vi "Robot Main.vi"() -> ()   [LabVIEW 2019]
doc: "This VI implements the framework and scheduler for your robotics program. It should not be necessary to modify the framework. You are expected to add your code to the VIs called from Robot Main - the ones located in the Team Code folder within the project."
uses:
  <vilib>/Rock Robotics/SystemInterfaces/i2clib/i2c_bus.ctl
panel:
  out "Normalized \nMeasured\nColor":cluster{"R":dbl, "G":dbl, "B":dbl}
  in  "UpdateColors":bool
  in  "Update Blue \nCalibration":cluster{"R":dbl, "G":dbl, "B":dbl}={"R"=0.143, "G"=0.427, "B"=0.429}
  in  "Update Green \nCalibration":cluster{"R":dbl, "G":dbl, "B":dbl}={"R"=0.197, "G"=0.561, "B"=0.24}
  in  "Update Red \nCalibration":cluster{"R":dbl, "G":dbl, "B":dbl}={"R"=0.561, "G"=0.323, "B"=0.114}
  in  "Update Yellow \nCalibration":cluster{"R":dbl, "G":dbl, "B":dbl}={"R"=0.361, "G"=0.524, "B"=0.113}
  out "Matched Color Name":string
  out "Match Confidence":dbl
  out "Measured Color":cluster{"R":dbl, "G":dbl, "B":dbl}
  in  "Init Blue \nCalibration":cluster{"R":dbl, "G":dbl, "B":dbl}={"R"=0.143, "G"=0.427, "B"=0.429}
  in  "Init Green \nCalibration":cluster{"R":dbl, "G":dbl, "B":dbl}={"R"=0.197, "G"=0.561, "B"=0.24}
  in  "Init Red \nCalibration":cluster{"R":dbl, "G":dbl, "B":dbl}={"R"=0.561, "G"=0.323, "B"=0.114}
  in  "Init Yellow \nCalibration":cluster{"R":dbl, "G":dbl, "B":dbl}={"R"=0.361, "G"=0.524, "B"=0.113}
  out "error out":errorcluster
  out "Proximity":u16(graph)
  out "Color":u32(colorbox)
  in  "I2C Bus":T1
  in  "Finish":bool
  # "Set These Items before running\nprogram"
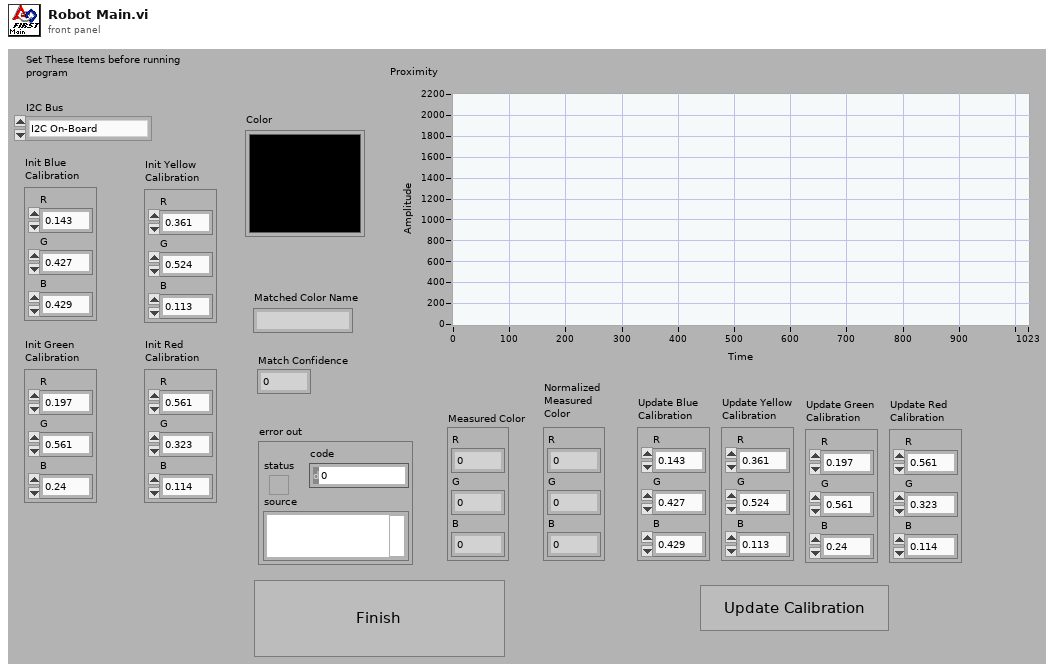
[diagram p1: front panel]
types:
  T1 = typedef "i2c_bus.ctl" = enum16{"I2C On-Board", "I2C MXP", "Invalid"}
  T2 = typedef "Color Sensor V3 DevRef.ctl" = cluster{"I2CDevRef":T3}
  T3 = typedef "WPI_I2CDevRef.ctl" = cluster{"DevStatus":errorcluster, "Device Address":u8, "Handle":i32, "I2C Bus":T1}
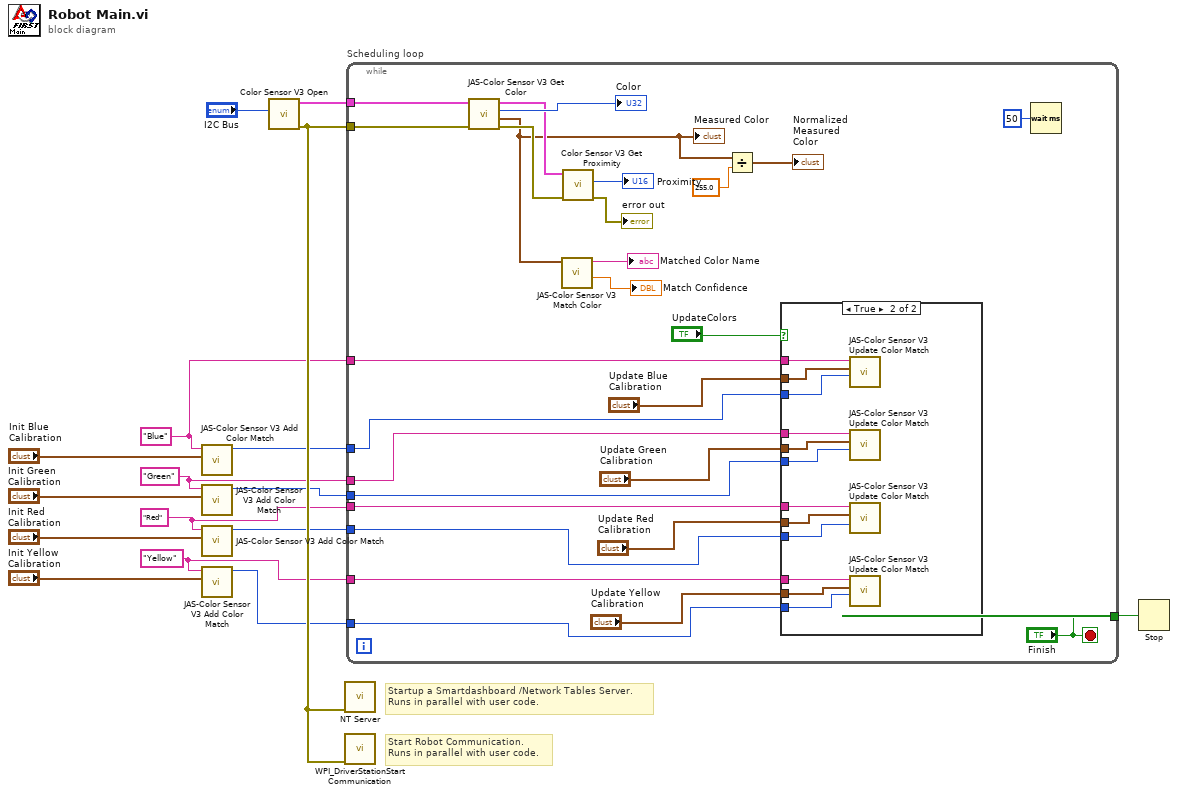
[diagram p0: block diagram]
diagram:
  w4 = "Yellow" ("Name")
  w5 = "Red" ("Name")
  w6 = "Green" ("Name")
  w7 = "Blue" ("Name")
  # "Startup a Smartdashboard /Network Tables Server.\nRuns in parallel with user code."
  # "Start Robot Communication.\nRuns in parallel with user code."
  n1 = call "JAS-Color Sensor V3 Add Color Match.vi"("Color"="Init Blue \nCalibration", "Name"=w7) -> ("ColorIndex"=w8:i32)  [unwired: 9 in]
  n2 = call "JAS-Color Sensor V3 Add Color Match.vi"("Color"="Init Green \nCalibration", "Name"=w6) -> ("ColorIndex"=w3:i32)  [unwired: 9 in]
  n3 = call "JAS-Color Sensor V3 Add Color Match.vi"("Color"="Init Red \nCalibration", "Name"=w5) -> ("ColorIndex"=w2:i32)  [unwired: 9 in]
  n4 = call "JAS-Color Sensor V3 Add Color Match.vi"("Color"="Init Yellow \nCalibration", "Name"=w4) -> ("ColorIndex"=w1:i32)  [unwired: 9 in]
  n5 = call <vilib>:"Color Sensor V3 Open.vi"("I2C Bus"="I2C Bus") -> ("error out"=w14:errorcluster, "ColorSensorDevRef"=w15:T2)  [unwired: 9 in]
  n6 = call <vilib>:"NT Server.vi"("error in (no error)"=w14) -> ()  [unwired: 11 in]
  n7 = call <vilib>:"WPI_DriverStationStart Communication.vi"("error in (no error)"=w14) -> ()  [unwired: 1 in, 10 out]
  n8 = while "Scheduling loop" {
    tunnel: w15 -> [w36]
    tunnel: w14 -> [w35]
    tunnel: ["Finish"] -> w13
    tunnel: w8 -> [w22]
    tunnel: w7 -> [w28]
    tunnel: w6 -> [w26]
    tunnel: w5 -> [w24]
    tunnel: w4 -> [w23]
    tunnel: w3 -> [w21]
    tunnel: w2 -> [w19]
    tunnel: w1 -> [w18]
    stop <- "Finish" stop-if-true
    n9 = call "JAS-Color Sensor V3 Get Color.vi"("error in (no error)"=w35, "ColorSensorDevRef"=w36) -> ("error out"=w41:errorcluster, "Normalized Color"=w32:cluster{"R":dbl, "G":dbl, "B":dbl}, "Color"=→"Color":u32, "ColorSensorDevRef out"=w40:T2)  [unwired: 6 in]
    "Measured Color" <- w32
    n10 = call "JAS-Color Sensor V3 Match Color.vi"("Measured Color"=w32) -> ("Confidence"=→"Match Confidence":dbl, "Matched Color Name"=→"Matched Color Name":string)  [unwired: 8 in, 1 out]
    n11 = call <vilib>:"Color Sensor V3 Get Proximity.vi"("error in (no error)"=w41, "ColorSensorDevRef"=w40) -> ("error out"=→"error out":errorcluster, "Proximity"=→"Proximity":u16)  [unwired: 7 in, 1 out]
    n12 = Divide(x=w32, y=255.0) -> (x/y=→"Normalized \nMeasured\nColor":cluster{"R":dbl, "G":dbl, "B":dbl})
    n13 = case shown="True" "UpdateColors" {
      tunnel: w28 -> [_ w55]
      tunnel: "Update Blue \nCalibration" -> [_ w54]
      tunnel: w26 -> [_ w53]
      tunnel: "Update Green \nCalibration" -> [_ w52]
      tunnel: w24 -> [_ w51]
      tunnel: w23 -> [_ w50]
      tunnel: w22 -> [_ w49]
      tunnel: w21 -> [_ w48]
      tunnel: "Update Red \nCalibration" -> [_ w47]
      tunnel: w19 -> [_ w46]
      tunnel: w18 -> [_ w44]
      tunnel: "Update Yellow \nCalibration" -> [_ w45]
      frame False {
      }
      frame True {
        n14 = call "JAS-Color Sensor V3 Update Color Match.vi"("ColorIndex"=w49, "Color"=w54, "Name"=w55) -> ()  [unwired: 9 in]
        n15 = call "JAS-Color Sensor V3 Update Color Match.vi"("ColorIndex"=w48, "Color"=w52, "Name"=w53) -> ()  [unwired: 9 in]
        n16 = call "JAS-Color Sensor V3 Update Color Match.vi"("ColorIndex"=w46, "Color"=w47, "Name"=w51) -> ()  [unwired: 9 in]
        n17 = call "JAS-Color Sensor V3 Update Color Match.vi"("ColorIndex"=w44, "Color"=w45, "Name"=w50) -> ()  [unwired: 9 in]
      }
    }
    n18 = Wait (ms)(milliseconds to wait=u32 50) -> ()  [unwired: 1 out]
  }
  n19 = Stop(stop? (T)=w13) -> ()
